vi "Read Is OK.vi"(8 "Error In":errorcluster, 11 "Writer In":refnum<class "Writer.lvclass">) -> (0 "Error Out":errorcluster, 2 "OK":bool, 3 "Writer Out":refnum<class "Writer.lvclass">)   [LabVIEW 2019, in "LabPack.lvlib" / "Writer.lvclass"]
doc: "Check if the internal encoder is OK."
uses:
  Writer.lvclass
  Writer.lvclass/Writer.ctl
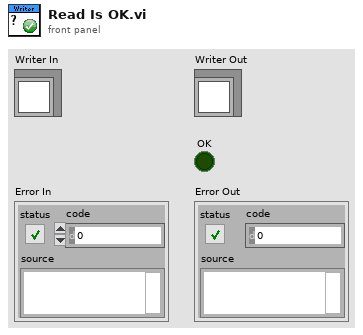
[diagram p1: front panel]
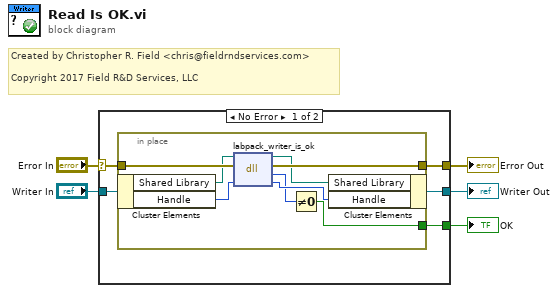
[diagram p0: block diagram]
diagram:
  # "Created by Christopher R. Field <chris@fieldrndservices.com>\n\nCopyright 2017 Field R&D Services, LLC"
  n1 = case shown="No Error" "Error In" {
    selector: "Error In" -> [w10 w19]
    tunnel: "Writer In" -> [w8 w20]
    tunnel: [w7 w20] -> w3
    tunnel: [w9 w19] -> w2
    tunnel: [w6 _] -> w1
    frame No Error {
      n2 = in-place {
        in-place-border: w10 -> [w18]
        in-place-border: [w17] -> w9
        in-place-border: [w11] -> w6
        n3 = in-place-cluster #1(w8) -> ("Shared Library"=w14:path, "Handle"=w16:u64)
        n4 = dll-call lib="D:/Users/cfield/Code/MessagePack/LabPack/LabVIEW/trunk/src/LabPack/Private/labpack-x64.dll" fn="labpack_writer_is_ok"(path in=w14, error in=w18, "writer"=w16) -> (path out=w13:path, error out=w17:errorcluster, "return type"=w12:i32, "writer"=w15:u64)  [unwired: 1 in]
        n5 = Not Equal To 0?(x=w12) -> (x != 0?=w11:bool)
        n6 = in-place-cluster #1("Shared Library"=w13, "Handle"=w15) -> (w7:refnum<class "Writer.lvclass">)
      }
    }
    frame Error {
    }
  }
  "Writer Out" <- w3
  "Error Out" <- w2
  "OK" <- w1
